vi "Read All UI.vi"(8 "error in (no error)":errorcluster, 11 "User Console in":refnum<class "User Console.lvclass">) -> (0 "error out":errorcluster, 3 "User Console out":refnum<class "User Console.lvclass">)   [LabVIEW 2019, in "User Console Actor.lvlib" / "User Console.lvclass"]
uses:
  User Console.lvclass
  Abstract User Console Actor/Abstract User Console Actor/Abstract User Console.lvclass
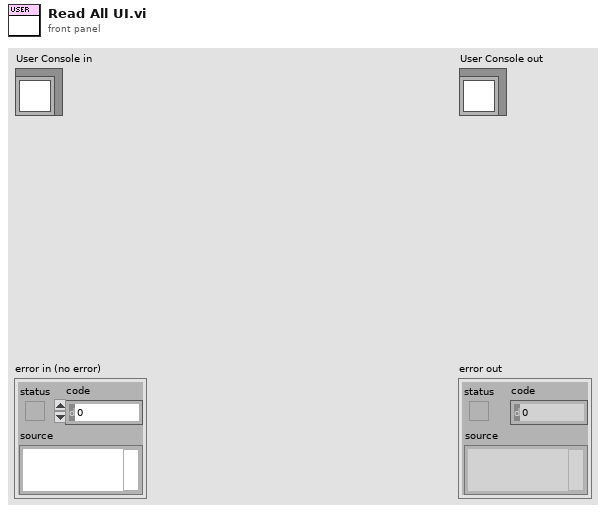
[diagram p1: front panel]
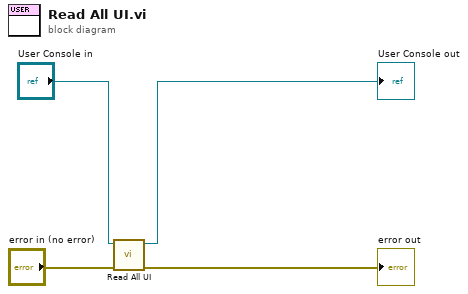
[diagram p0: block diagram]
diagram:
  n1 = call-parent "Read All UI.vi"("error in (no error)"="error in (no error)", "Abstract User Console in"="User Console in") -> ("error out"=→"error out":errorcluster, "Abstract User Console out"=→"User Console out":refnum<class "User Console.lvclass">)  [unwired: 8 in]
